vi "WriteXMLToFile.vi"(8 "error in (no error)":errorcluster, 10 "Node Ptr":u64, 11 "selected path":path) -> (0 "error out":errorcluster)   [LabVIEW 2024, in "Embedded TDMS Logger System Explorer.lvlib"]
doc: "Writes the current Custom Device configuration to XML format"
uses:
  Embedded TDMS Logger System Explorer.lvlib
  Shared/File Classes/File/File.lvclass
  NationalInstruments.VeriStand.SystemDefinitionAPI
  <vilib>/NI VeriStand/Custom Device API/Custom Device API.lvlib
  Shared/SegmentOptions.ctl
  Shared/Segmentation.ctl
  Shared/Embedded TDMS Logger Shared.lvlib
  <vilib>/NI VeriStand/Custom Device API/Get Item Property (Boolean).vi
  <vilib>/NI VeriStand/Custom Device API/Get Item Property (Double).vi
  <vilib>/NI VeriStand/Custom Device API/Get Item Property (U16).vi
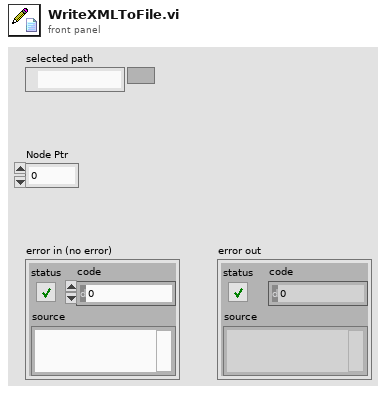
[diagram p1: front panel]
types:
  T1 = typedef "Embedded TDMS Logger Shared.lvlib/Segmentation.ctl" = cluster{"Segment":bool, "Segment Every":dbl, "Segment by":T2}
  T2 = typedef "SegmentOptions.ctl" = enum16{"Time (s)", "Size (MB)"}
  T3 = enum16{"open", "replace", "create", "open or create", "replace or create", "replace or create with confirmation"}
  T4 = typedef "Custom Device API.lvlib/Custom Device Pointer.ctl" = refnum<k24>
  T5 = typedef "Custom Device API.lvlib/Custom Device Item Ref.ctl" = u64
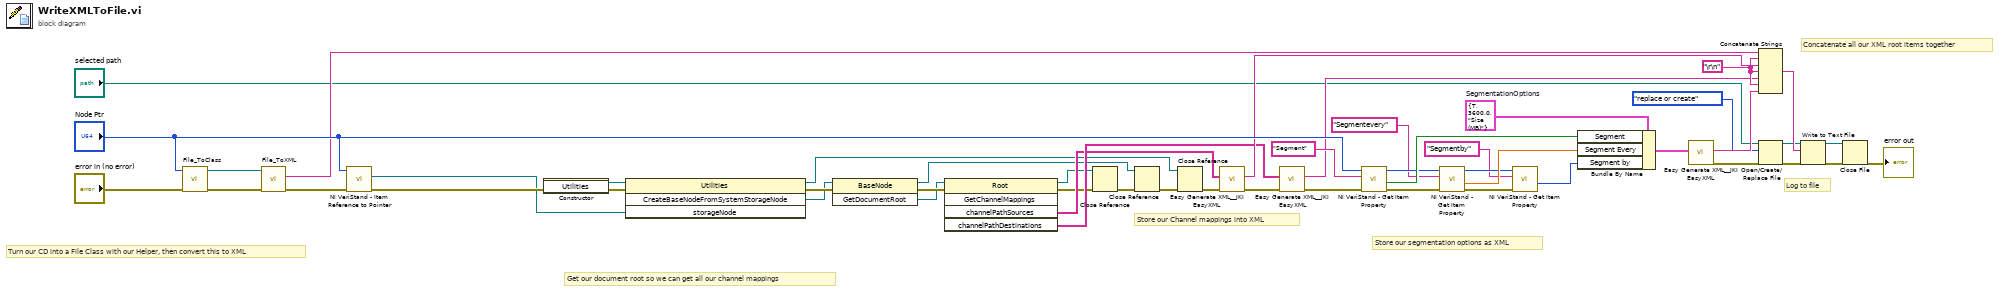
[diagram p0: block diagram]
diagram:
  w35 = T1 {"Segment"=TRUE, "Segment Every"=3600.0, "Segment by"=enum."Size (MB)"}  # SegmentationOptions
  w34 = "\r\n"
  # "Log to file"
  # "Concatenate all our XML root items together"
  # "Store our segmentation options as XML"
  # "Store our Channel mappings into XML"
  # "Get our document root so we can get all our channel mappings"
  # "Turn our CD into a File Class with our Helper, then convert this to XML"
  n1 = call "File_ToClass.vi"("error in (no error)"="error in (no error)", "Item Ref in"="Node Ptr") -> ("error out"=w33:errorcluster, "File out"=w2:refnum<class "File.lvclass">)  [unwired: 7 in, 1 out]
  n2 = call-dynamic "File_ToXML.vi"("error in (no error)"=w33, "File in"=w2) -> ("error out"=w14:errorcluster, "XML String"=w24:string)  [unwired: 7 in, 1 out]
  n3 = call <vilib>:"NI VeriStand - Item Reference to Pointer.vi"("error in (no error)"=w14, "Item Ref in"="Node Ptr") -> ("error out"=w25:errorcluster, "Node Pointer"=w13:T4)  [unwired: 6 in, 2 out]
  n4 = constructor class="Utilities"(error in=w25) -> (reference out=w9:refnum<k24>, error out=w10:errorcluster)  [unwired: 2 in, 1 out]
  n5 = invoke class="Utilities" method="CreateBaseNodeFromSystemStorageNode"(reference=w9, error in=w10, "storageNode"=w13) -> (reference out=w20:refnum<k24>, error out=w12:errorcluster, "CreateBaseNodeFromSystemStorageNode"=w11:refnum<k24>)  [unwired: 1 in, 1 out]
  n6 = invoke class="BaseNode" method="GetDocumentRoot"(reference=w11, error in=w12) -> (reference out=w19:refnum<k24>, error out=w16:errorcluster, "GetDocumentRoot"=w15:refnum<k24>)  [unwired: 1 in]
  n7 = invoke class="Root" method="GetChannelMappings"(reference=w15, error in=w16) -> (reference out=w21:refnum<k24>, error out=w22:errorcluster, "channelPathSources"=w28:string[], "channelPathDestinations"=w29:string[])  [unwired: 3 in, 1 out]
  n8 = Close Reference(reference=w21, error in (no error)=w22) -> (error out=w17:errorcluster)
  n9 = Close Reference(reference=w19, error in (no error)=w17) -> (error out=w18:errorcluster)
  n10 = Close Reference(reference=w20, error in (no error)=w18) -> (error out=w23:errorcluster)
  n11 = call <vilib>:"Easy Generate XML__JKI EasyXML.vi"("error in (no error)"=w23, "LabVIEW Data"=w28) -> ("error out"=w30:errorcluster, "XML String"=w32:string)  [unwired: 8 in]
  n12 = call <vilib>:"Easy Generate XML__JKI EasyXML.vi"("error in (no error)"=w30, "LabVIEW Data"=w29) -> ("error out"=w39:errorcluster, "XML String"=w31:string)  [unwired: 8 in]
  n13 = call-poly <vilib>:"NI VeriStand - Get Item Property.vi"("error in (no error)"=w39, "Property Name"="Segment", "Item Ref in"="Node Ptr") -> ("error out"=w47:errorcluster, "Value"=w49:bool, "Item Ref out"=w46:T5)  [unwired: 5 in, 1 out]
  n14 = call-poly <vilib>:"NI VeriStand - Get Item Property.vi"("error in (no error)"=w47, "Property Name"="Segmentevery", "Item Ref in"=w46) -> ("error out"=w48:errorcluster, "Value"=w50:dbl, "Item Ref out"=w45:T5)  [unwired: 5 in, 1 out]
  n15 = call-poly <vilib>:"NI VeriStand - Get Item Property.vi"("error in (no error)"=w48, "Property Name"="Segmentby", "Item Ref in"=w45) -> ("Value"=w44:u16)  [unwired: 5 in, 3 out]
  n16 = Bundle By Name(cluster=w35, "Segment"=w49, "Segment Every"=w50, "Segment by"=w44) -> (w38:T1)
  n17 = call <vilib>:"Easy Generate XML__JKI EasyXML.vi"("LabVIEW Data"=w38) -> ("error out"=w37:errorcluster, "XML String"=w36:string)  [unwired: 9 in]
  n18 = Concatenate Strings(w24, w34, w32, w34, w31, w34, w36) -> (w26:string)
  n19 = Open/Create/Replace File(file path (use dialog)="selected path", error in=w37, operation (0:open)=T3."replace or create") -> (refnum out=w4:refnum<file>, error out=w6:errorcluster)  [unwired: 3 in, 1 out]
  n20 = Write to Text File(file (use dialog)=w4, text=w26, error in=w6) -> (refnum out=w7:refnum<file>, error out=w8:errorcluster)  [unwired: 1 in, 1 out]
  n21 = Close File(refnum=w7, error in=w8) -> (error out=→"error out":errorcluster)  [unwired: 1 out]
